vi "GetIntakeQueue.vi"() -> (3 "queue out":refnum<queue>)   [LabVIEW 2015]
uses:
  Typedef/IntakeControllerMsg.ctl
  Typedef/IntakeControllerActions.ctl
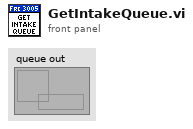
[diagram p1: front panel]
types:
  T1 = typedef "IntakeControllerMsg.ctl" = cluster{"Cmd":T2, "Data":variant}
  T2 = typedef "IntakeControllerActions.ctl" = enum16{"Wait on Intake Rear", "Wait on Angle Rear", "Go To Angle Rear", "Wait on Intake Front", "Wait on Angle Front", "Set Roller Front", "Set Roller Rear", "Go To Angle Front", "Wait ms"}
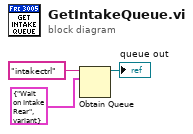
[diagram p0: block diagram]
diagram:
  n1 = Obtain Queue(name (unnamed)="intakectrl", element data type=T1 {"Cmd"=enum."Wait on Intake Rear", "Data"=variant}) -> (queue out=→"queue out":refnum<queue>)  [unwired: 3 in, 2 out]
